vi "LJM logger program config string to array.vi"(5 "Delimiter (#!#)":string="#!#", 7 "Max Num Elements":i32=100, 8 "Int Config String In":string, 9 "Bool Config String In":string, 10 "String Config String In 2":string, 11 "String Config String In":string) -> (0 "Int Config Array Out":i32[](array[numeric]), 1 "Bool Config Array Out":bool[](array[boolean]), 2 "String Config Array Out 2":string[](array[string]), 3 "String Config Array Out":string[](array[string]))   [LabVIEW 2026]
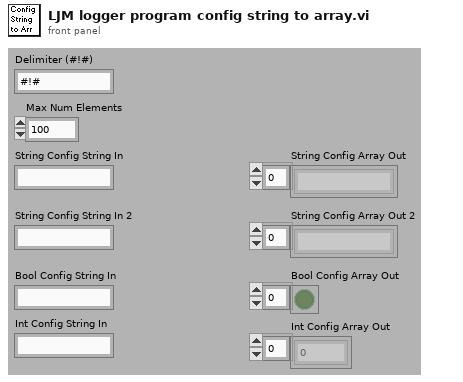
[diagram p1: front panel]
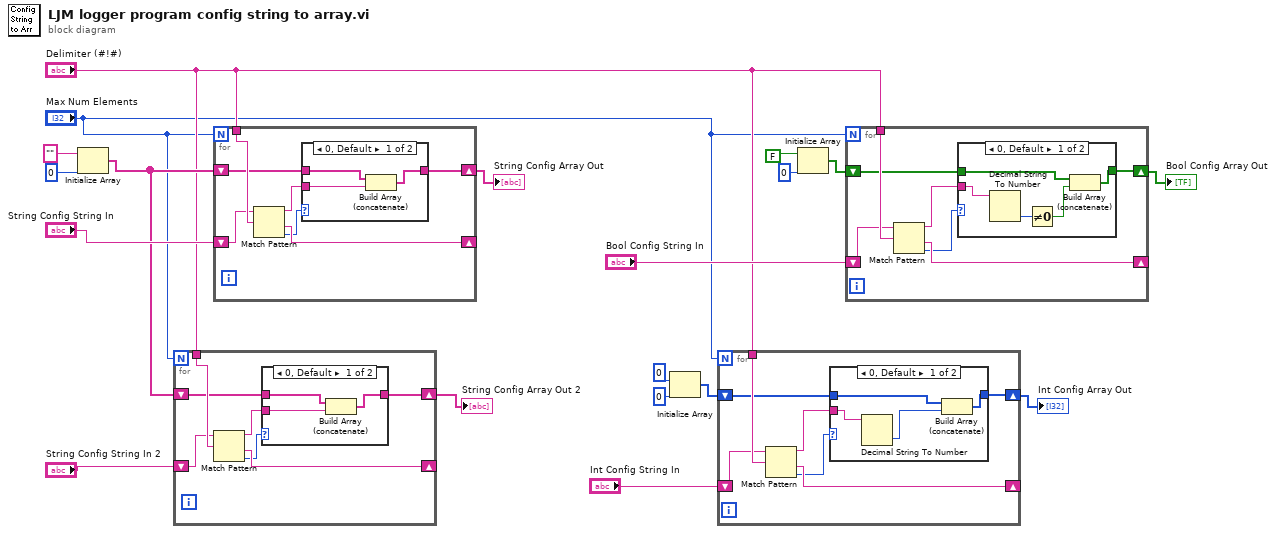
[diagram p0: block diagram]
diagram:
  n1 = Initialize Array("" ("String Config String In"), 0 ("dimension size")) -> (w9:string[])
  n2 = for {
    N: "Max Num Elements" -> [_]
    shift-right: [w24] -> _
    shift-left: "String Config String In 2" -> [w25]
    tunnel: "Delimiter (#!#)" -> [w26]
    shift-right: [w22] -> w10
    shift-left: w9 -> [w21]
    n3 = Match Pattern(string=w25, regular expression=w26) -> (before substring=w20:string, after substring=w24:string, offset past match=w23:i32)  [unwired: 1 in, 1 out]
    n4 = case shown="0, Default" w23 {
      tunnel: w20 -> [w28 _]
      tunnel: [w27 w30] -> w22
      tunnel: w21 -> [w29 w30]
      frame 0, Default {
        n5 = Build Array (concatenate)(w29, w28) -> (w27:string[])
      }
      frame -1 {
        # "No more matches"
      }
    }
  }
  "String Config Array Out 2" <- w10
  n6 = for {
    N: "Max Num Elements" -> [_]
    shift-right: [w35] -> _
    shift-left: "String Config String In" -> [w36]
    tunnel: "Delimiter (#!#)" -> [w37]
    shift-right: [w33] -> w11
    shift-left: w9 -> [w32]
    n7 = Match Pattern(string=w36, regular expression=w37) -> (before substring=w31:string, after substring=w35:string, offset past match=w34:i32)  [unwired: 1 in, 1 out]
    n8 = case shown="0, Default" w34 {
      tunnel: w31 -> [w39 _]
      tunnel: [w38 w41] -> w33
      tunnel: w32 -> [w40 w41]
      frame 0, Default {
        n9 = Build Array (concatenate)(w40, w39) -> (w38:string[])
      }
      frame -1 {
        # "No more matches"
      }
    }
  }
  "String Config Array Out" <- w11
  n10 = Initialize Array(0 ("dimension size"), 0 ("dimension size")) -> (w5:i32[])
  n11 = for {
    N: "Max Num Elements" -> [_]
    shift-right: [w46] -> _
    shift-left: "Int Config String In" -> [w47]
    tunnel: "Delimiter (#!#)" -> [w48]
    shift-right: [w44] -> w3
    shift-left: w5 -> [w43]
    n12 = Match Pattern(string=w47, regular expression=w48) -> (before substring=w45:string, after substring=w46:string, offset past match=w42:i32)  [unwired: 1 in, 1 out]
    n13 = case shown="0, Default" w42 {
      tunnel: w45 -> [w50 _]
      tunnel: [w52 w53] -> w44
      tunnel: w43 -> [w51 w53]
      frame 0, Default {
        n14 = Decimal String To Number(string=w50) -> (number=w49:i32)  [unwired: 2 in, 1 out]
        n15 = Build Array (concatenate)(w51, w49) -> (w52:i32[])
      }
      frame -1 {
        # "No more matches"
      }
    }
  }
  "Int Config Array Out" <- w3
  n16 = Initialize Array(FALSE, 0 ("dimension size")) -> (w13:bool[])
  n17 = for {
    N: "Max Num Elements" -> [_]
    shift-right: [w58] -> _
    shift-left: "Bool Config String In" -> [w59]
    tunnel: "Delimiter (#!#)" -> [w60]
    shift-right: [w56] -> w12
    shift-left: w13 -> [w55]
    n18 = Match Pattern(string=w59, regular expression=w60) -> (before substring=w57:string, after substring=w58:string, offset past match=w54:i32)  [unwired: 1 in, 1 out]
    n19 = case shown="0, Default" w54 {
      tunnel: w57 -> [w63 _]
      tunnel: [w65 w66] -> w56
      tunnel: w55 -> [w64 w66]
      frame 0, Default {
        n20 = Decimal String To Number(string=w63) -> (number=w62:i32)  [unwired: 2 in, 1 out]
        n21 = Not Equal To 0?(x=w62) -> (x != 0?=w61:bool)
        n22 = Build Array (concatenate)(w64, w61) -> (w65:bool[])
      }
      frame -1 {
        # "No more matches"
      }
    }
  }
  "Bool Config Array Out" <- w12
